vi "Initialise Front Panel.vi"(7 "This VI":refnum<vi>, 11 "UI Ref":T1) -> (0 "error out":errorcluster)   [LabVIEW 2021]
uses:
  Controls/UI References.ctl
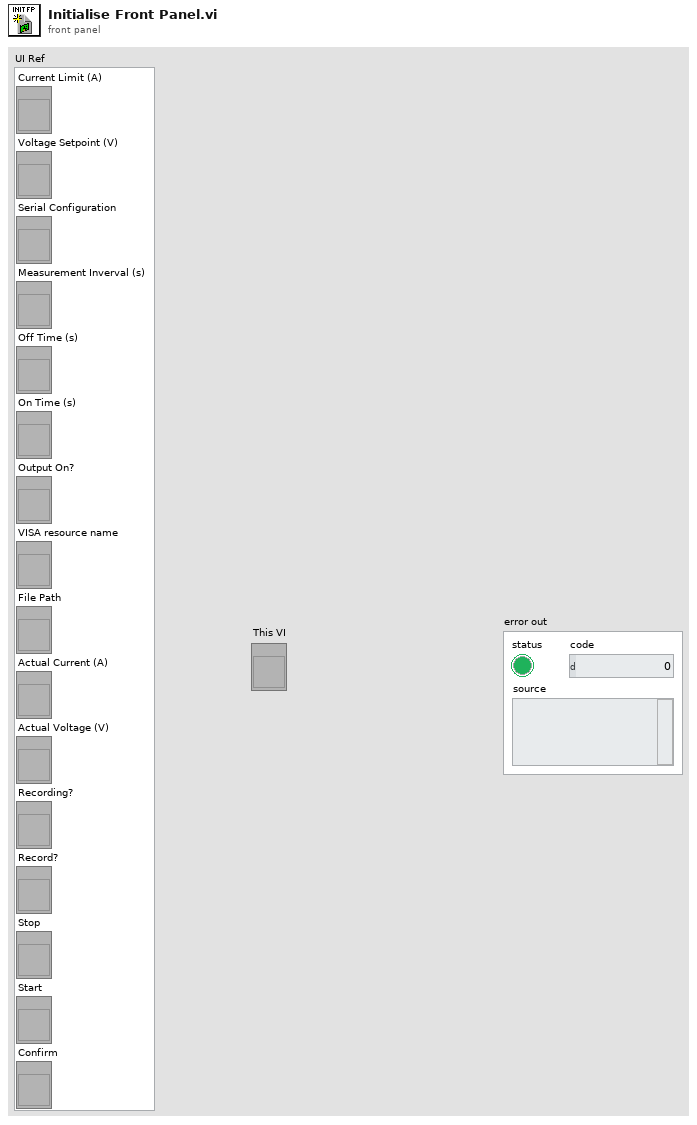
[diagram p1: front panel]
types:
  T1 = typedef "UI References.ctl" = cluster{"Current Limit (A)":refnum<vi>, "Voltage Setpoint (V)":refnum<vi>, "Serial Configuration":refnum<vi>, "Measurement Inverval (s)":refnum<vi>, "Off Time (s)":refnum<vi>, "On Time (s)":refnum<vi>, "Output On?":refnum<vi>, "VISA resource name":refnum<vi>, "File Path":refnum<vi>, "Actual Current (A)":refnum<vi>, "Actual Voltage (V)":refnum<vi>, "Recording?":refnum<vi>, "Record?":refnum<vi>, "Stop":refnum<vi>, "Start":refnum<vi>, "Confirm":refnum<vi>}
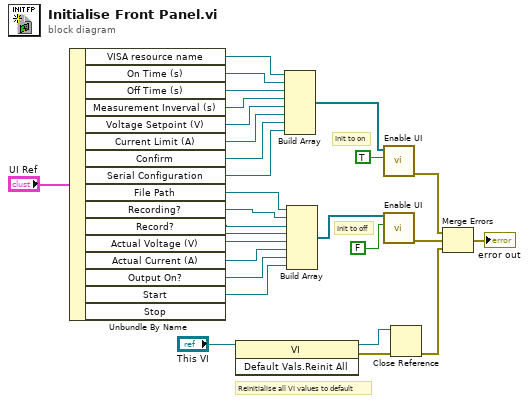
[diagram p0: block diagram]
diagram:
  # "Init to on"
  # "Init to off"
  # "Reinitialise all VI values to default"
  n1 = Unbundle By Name("UI Ref") -> ("VISA resource name"=w2:refnum<vi>, "On Time (s)"=w1:refnum<vi>, "Off Time (s)"=w17:refnum<vi>, "Measurement Inverval (s)"=w16:refnum<vi>, "Voltage Setpoint (V)"=w15:refnum<vi>, "Current Limit (A)"=w14:refnum<vi>, "Confirm"=w13:refnum<vi>, "Serial Configuration"=w12:refnum<vi>, "File Path"=w5:refnum<vi>, "Recording?"=w4:refnum<vi>, "Record?"=w3:refnum<vi>, "Actual Voltage (V)"=w11:refnum<vi>, "Actual Current (A)"=w10:refnum<vi>, "Output On?"=w9:refnum<vi>, "Start"=w8:refnum<vi>)  [unwired: 1 out]
  n2 = invoke class="VI" method="Default Vals.Reinit All"(reference="This VI") -> (reference out=w26:refnum<vi>, error out=w23:errorcluster)  [unwired: 2 in, 1 out]
  n3 = Build Array(w2, w1, w17, w16, w15, w14, w13, w12) -> (w6:refnum<vi>[])
  n4 = Build Array(w5, w4, w3, w3, w11, w10, w9, w8) -> (w7:refnum<vi>[])
  n5 = call "Enable UI.vi"("Enable?"=TRUE, "output cluster"=w6) -> ("error out"=w22:errorcluster)  [unwired: 9 in]
  n6 = call "Enable UI.vi"("Enable?"=FALSE, "output cluster"=w7) -> ("error out"=w21:errorcluster)  [unwired: 9 in]
  n7 = Close Reference(reference=w26, error in (no error)=w23) -> (error out=w20:errorcluster)
  n8 = Merge Errors(w22, w21, w20) -> (→"error out":errorcluster)
